vi "Match from String Arr.vi"(7 "Ignore case (TRUE def)":bool=TRUE, 10 "String to match":string="c:\\DATA", 11 "String Array In":string[](array[string])=["the settings file open properly", "Init", "the temperature file open properly", "astrocamInit: lodFile = C:\\vlt\\assembly\\h2rg-20141010\\SNAP\\tim_h2rg_SNAP.lod", "Getting device bindings ... done !", "Opening PCI driver ... ", "done!", "Calling astrocamConfig ", "astrocamConfig start ...", "Setting up controllerdone!", "Opening shutter ...", "Configuring ...", "RNT = 1", "OFA 0x1ec", "Waiting for image ..", "Done=true ", "GotImage - returning  ", "c:\\DATA\\20141011-102717-0.fits", "Got image.", "Waiting for image ..", "Done=true ", "GotImage - returning  ", "c:\\DATA\\20141011-102717-1.fits", "Got image.", "Close", "Test", "Done", ""]) -> (1 "Inx Exact match":i32[](array[numeric]), 2 "Inx matches":i32[](array[numeric]), 3 "String Array Matched":string[](array[string])=["c:\\DATA\\20141011-102717-0.fits", "c:\\DATA\\20141011-102717-1.fits"], 5 "Str found?":bool)   [LabVIEW 2024]
uses:
  <vilib>/Utility/error.llb/Trim Whitespace One-Sided.vi
panel:
  out "Array Size":i32=2
  out "String Found Inx":i32[](array[numeric])=[-1, -1, -1, -1, -1, -1, -1, -1, -1, -1, -1, -1, -1, -1, -1, -1, -1, 0, -1, -1, -1, -1, 0, -1, -1, -1, -1, -1]
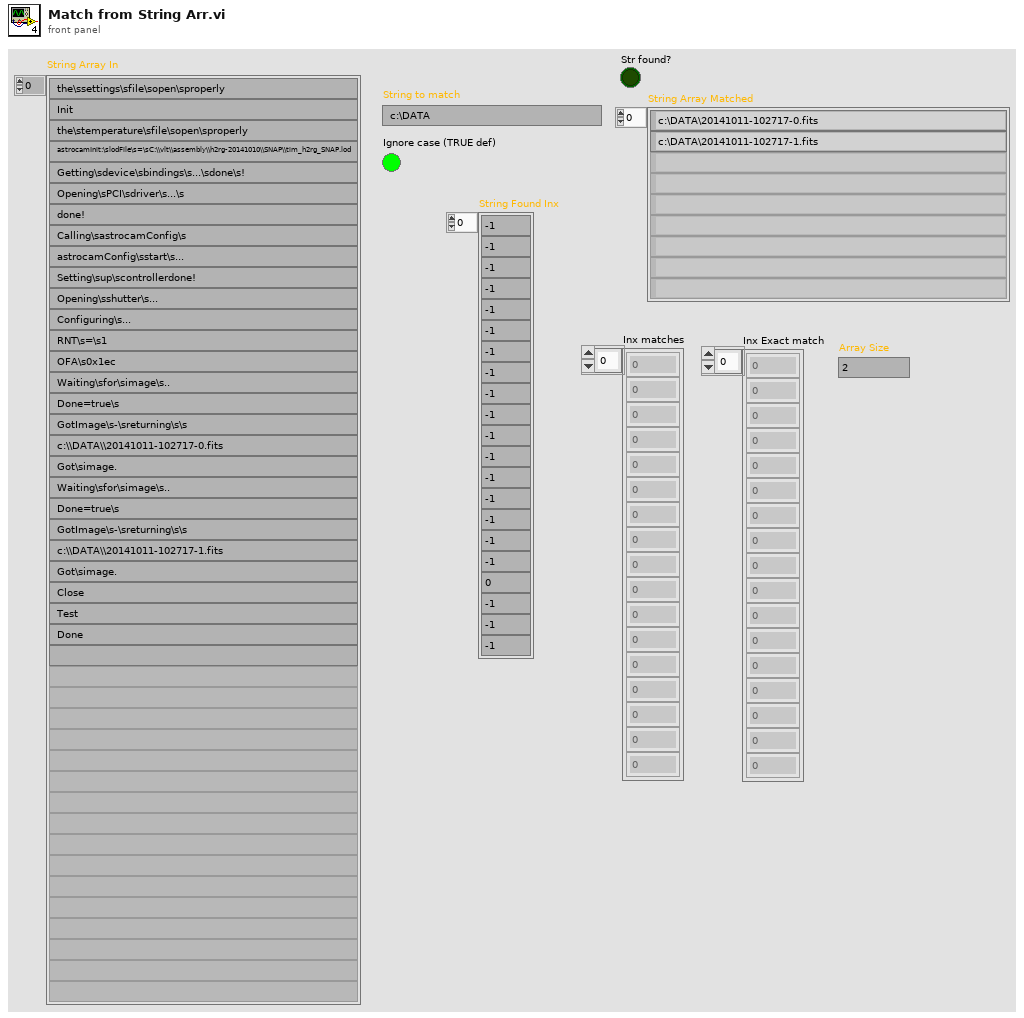
[diagram p1: front panel]
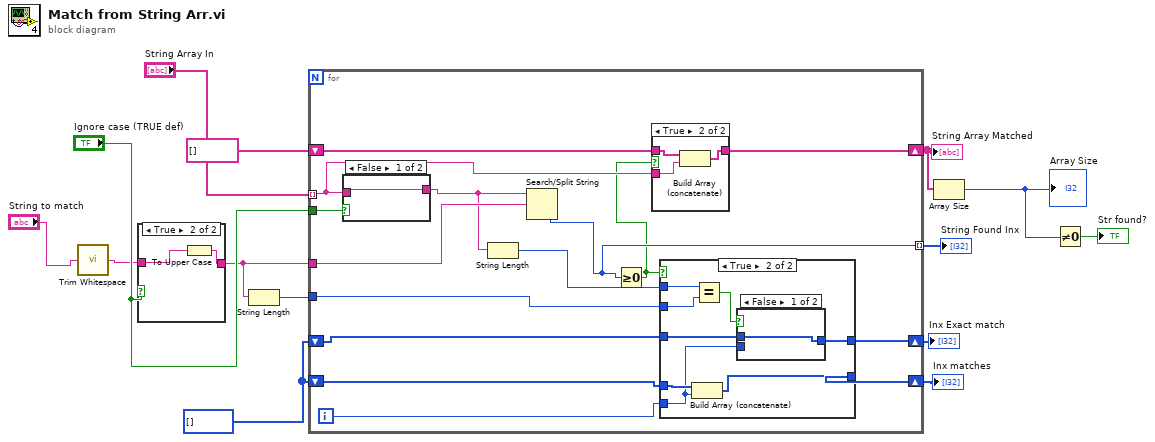
[diagram p0: block diagram]
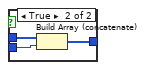
[diagram p4: hidden frame]
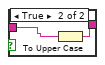
[diagram p5: hidden frame]
diagram:
  w4 = i32[] []
  n1 = call <vilib>:"Trim Whitespace.vi"("string"="String to match") -> ("trimmed string"=w8:string)  [unwired: 1 in]
  n2 = case shown="True" "Ignore case (TRUE def)" {
    tunnel: w8 -> [w15 w17]
    tunnel: [w15 w16] -> w7
    frame False {
    }
    frame True {
      n3 = To Upper Case(1:w17) -> (0:w16:string)
    }
  }
  n4 = String Length(string=w7) -> (length=w6:i32)
  n5 = for {
    tunnel: "String Array In" -> [w29] mode=indexing
    shift-right: [w32] -> w12
    shift-left: string[] [] -> [w31]
    tunnel: [w30] -> w13 mode=indexing
    tunnel: "Ignore case (TRUE def)" -> [w28]
    tunnel: w7 -> [w27]
    shift-right: [w20] -> w5
    shift-left: w4 -> [w24]
    tunnel: w6 -> [w23]
    shift-right: [w18] -> w3
    shift-left: w4 -> [w19]
    i -> [w25]
    n6 = case shown="False" w28 {
      tunnel: w29 -> [w47 w49]
      tunnel: [w47 w48] -> w22
      frame False {
      }
      frame True {
        n7 = To Upper Case(1:w49) -> (0:w48:string)
      }
    }
    n8 = String Length(string=w22) -> (length=w21:i32)
    n9 = Search/Split String(string=w22, search string/char (-)=w27) -> (offset of match=w30:i32)  [unwired: 1 in, 2 out]
    n10 = Greater Or Equal To 0?(x=w30) -> (x >= 0?=w26:bool)
    n11 = case shown="True" w26 {
      tunnel: w29 -> [_ w53]
      tunnel: [w50 w52] -> w32
      tunnel: w31 -> [w50 w51]
      frame False {
      }
      frame True {
        n12 = Build Array (concatenate)(w51, w53) -> (w52:string[])
      }
    }
    n13 = case shown="True" w26 {
      tunnel: [w34 w42] -> w20
      tunnel: w24 -> [w34 w41]
      tunnel: w25 -> [_ w35]
      tunnel: w23 -> [_ w39]
      tunnel: w21 -> [_ w40]
      tunnel: w19 -> [w33 w37]
      tunnel: [w33 w36] -> w18
      frame False {
      }
      frame True {
        n14 = Build Array (concatenate)(w41, w35) -> (w42:i32[])
        n15 = Equal?(x=w40, y=w39) -> (x = y?=w38:bool)
        n16 = case shown="False" w38 {
          tunnel: w37 -> [w43 w46]
          tunnel: [w43 w45] -> w36
          tunnel: w35 -> [_ w44]
          frame False {
          }
          frame True {
            n17 = Build Array (concatenate)(w46, w44) -> (w45:i32[])
          }
        }
      }
    }
  }
  "String Array Matched" <- w12
  "String Found Inx" <- w13
  "Inx matches" <- w5
  "Inx Exact match" <- w3
  n18 = Array Size(array=w12) -> (size(s)=w2:i32)
  "Array Size" <- w2
  n19 = Not Equal To 0?(x=w2) -> (x != 0?=→"Str found?":bool)
